vi "pr650_display_blink.vi"(0 "error out 2":errorcluster, 1 "VISA resource name out 2":refnum<visa-resource-name>) -> (2 "error out":errorcluster, 3 "return count":u32, 4 "VISA resource name out":refnum<visa-resource-name>)   [LabVIEW 2010]
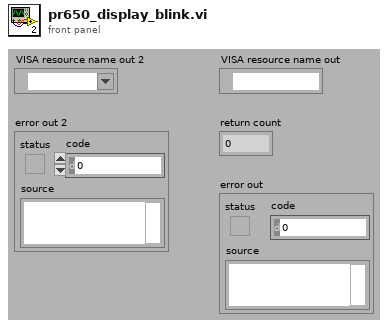
[diagram p1: front panel]
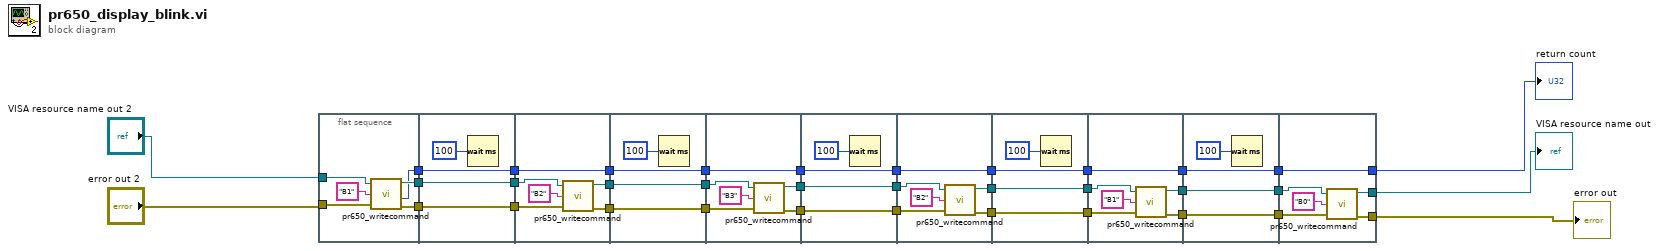
[diagram p0: block diagram]
diagram:
  n1 = flat-sequence {
    tunnel: "VISA resource name out 2" -> [w41]
    tunnel: "error out 2" -> [w40]
    tunnel: [w39] -> w35
    tunnel: [w38] -> w34
    tunnel: [w37] -> w33
    tunnel: w35 -> [w45]
    tunnel: w34 -> [w44]
    tunnel: w33 -> [w43]
    tunnel: [w45] -> w32
    tunnel: [w44] -> w31
    tunnel: [w43] -> w30
    tunnel: w32 -> [w48]
    tunnel: w31 -> [w51]
    tunnel: w30 -> [w49]
    tunnel: [w51] -> w29
    tunnel: [w46] -> w28
    tunnel: [w47] -> w27
    tunnel: w29 -> [w54]
    tunnel: w28 -> [w53]
    tunnel: w27 -> [w55]
    tunnel: [w55] -> w26
    tunnel: [w54] -> w25
    tunnel: [w53] -> w24
    tunnel: w26 -> [w59]
    tunnel: w25 -> [w61]
    tunnel: w24 -> [w58]
    tunnel: [w61] -> w23
    tunnel: [w57] -> w22
    tunnel: [w56] -> w21
    tunnel: w23 -> [w65]
    tunnel: [w65] -> w20
    tunnel: w22 -> [w63]
    tunnel: [w63] -> w19
    tunnel: w21 -> [w62]
    tunnel: [w62] -> w18
    tunnel: w20 -> [w71]
    tunnel: [w71] -> w17
    tunnel: w19 -> [w69]
    tunnel: w18 -> [w68]
    tunnel: [w67] -> w16
    tunnel: [w66] -> w15
    tunnel: w17 -> [w75]
    tunnel: [w75] -> w14
    tunnel: [w73] -> w13
    tunnel: w16 -> [w73]
    tunnel: [w72] -> w12
    tunnel: w15 -> [w72]
    tunnel: w14 -> [w81]
    tunnel: [w81] -> w11
    tunnel: w13 -> [w79]
    tunnel: w12 -> [w78]
    tunnel: [w77] -> w10
    tunnel: [w76] -> w9
    tunnel: w11 -> [w85]
    tunnel: [w85] -> w8
    tunnel: [w83] -> w7
    tunnel: w10 -> [w83]
    tunnel: w9 -> [w82]
    tunnel: [w82] -> w6
    tunnel: [w91] -> w3
    tunnel: w8 -> [w91]
    tunnel: w7 -> [w89]
    tunnel: w6 -> [w88]
    tunnel: [w87] -> w4
    tunnel: [w86] -> w5
    frame #0 {
      n2 = call "pr650_writecommand.vi"("error in"=w40, "write buffer"="B1", "VISA resource name in"=w41) -> ("error out"=w37:errorcluster, "return count"=w38:u32, "VISA resource name out"=w39:refnum<visa-resource-name>)  [unwired: 1 in]
    }
    frame #1 {
      n3 = Wait (ms)(milliseconds to wait=u32 100) -> ()  [unwired: 1 out]
    }
    frame #2 {
      n4 = call "pr650_writecommand.vi"("error in"=w49, "write buffer"="B2", "VISA resource name in"=w48) -> ("error out"=w46:errorcluster, "VISA resource name out"=w47:refnum<visa-resource-name>)  [unwired: 1 in, 1 out]
    }
    frame #3 {
      n5 = Wait (ms)(milliseconds to wait=u32 100) -> ()  [unwired: 1 out]
    }
    frame #4 {
      n6 = call "pr650_writecommand.vi"("error in"=w58, "write buffer"="B3", "VISA resource name in"=w59) -> ("error out"=w56:errorcluster, "VISA resource name out"=w57:refnum<visa-resource-name>)  [unwired: 1 in, 1 out]
    }
    frame #5 {
      n7 = Wait (ms)(milliseconds to wait=u32 100) -> ()  [unwired: 1 out]
    }
    frame #6 {
      n8 = call "pr650_writecommand.vi"("error in"=w68, "write buffer"="B2", "VISA resource name in"=w69) -> ("error out"=w66:errorcluster, "VISA resource name out"=w67:refnum<visa-resource-name>)  [unwired: 1 in, 1 out]
    }
    frame #7 {
      n9 = Wait (ms)(milliseconds to wait=u32 100) -> ()  [unwired: 1 out]
    }
    frame #8 {
      n10 = call "pr650_writecommand.vi"("error in"=w78, "write buffer"="B1", "VISA resource name in"=w79) -> ("error out"=w77:errorcluster, "VISA resource name out"=w76:refnum<visa-resource-name>)  [unwired: 1 in, 1 out]
    }
    frame #9 {
      n11 = Wait (ms)(milliseconds to wait=u32 100) -> ()  [unwired: 1 out]
    }
    frame #10 {
      n12 = call "pr650_writecommand.vi"("error in"=w89, "write buffer"="B0", "VISA resource name in"=w88) -> ("error out"=w86:errorcluster, "VISA resource name out"=w87:refnum<visa-resource-name>)  [unwired: 1 in, 1 out]
    }
  }
  "error out" <- w5
  "VISA resource name out" <- w4
  "return count" <- w3
